vi "ParameterSubUI.vi"() -> ()   [LabVIEW 2016]
uses:
  Package ResourceControl/ViHandler/ViHandler.ViInfo.ctl
  Package Libraries/Message Queue/private/MessageQueue.MessageTypeDef.ctl
  Package ResourceControl/ViHandler/ViHandler.RunModes.ctl
  Package ErrorHandling/ErrorHandling.lvclass/ErrorHandling.ctl
  Package ErrorHandling/ErrorHandling.checkForErrorAndHandle.vi
  Package ErrorHandling/ErrorHandling.GetErrorHandler.vi
  <vilib>/Utility/error.llb/Clear Errors.vi
  Package Libraries/StringFunctions/StringFunctions_ReplaceAllBlindSigns.vi
  <vilib>/dlg_ctls.llb/Space Constant.vi
  Package Simulation/Modell/Umgebung/Umgebung.ParameterUI.vi
  Package Simulation/Modell/Hausmodell/Hausmodell.ParameterUI.vi
  <vilib>/Utility/error.llb/Error Cluster From Error Code.vi
  Package Libraries/TimingFunctions/TimingFunctions_getUtcTimestamp.vi
  <vilib>/Utility/error.llb/Trim Whitespace.vi
  <vilib>/Utility/error.llb/Search and Replace Pattern.vi
  Package ErrorHandling/ErrorHandling.addLastErrorToFile.vi
  <vilib>/ErrorRing/Error Ring.xnode
  Package ErrorHandling/ErrorHandling.lvclass
  Package ResourceControl/ViHandler/ViHandler.lvclass
  Package Simulation/Modell/Hausmodell/Hausmodell.lvclass
  Package Simulation/Modell/Sondenmodell/Sondenmodell.lvclass
  Package Simulation/Modell/Umgebung/Umgebung.lvclass
panel:
  in  "UmgebungBtn":bool
  in  "WPBtn":bool
  in  "SondenBtn":bool
  in  "HausBtn":bool
  out "EndOfBuffer[ms]":u32
  out "ViInfoTemp":T1
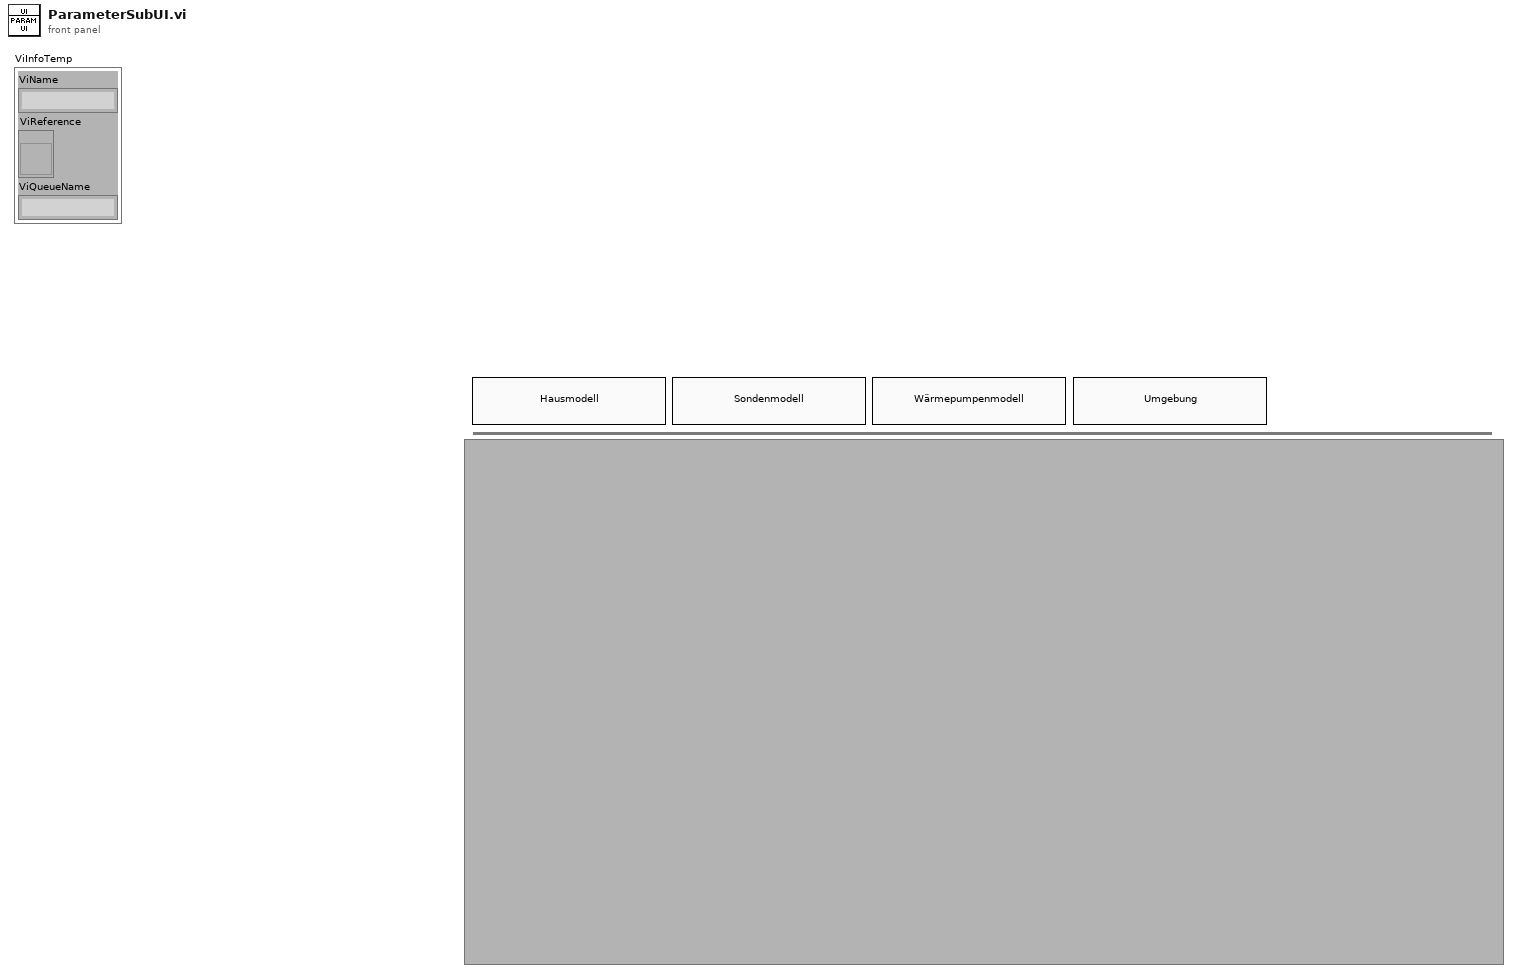
[diagram p1: front panel]
types:
  T1 = typedef "ViHandler.lvclass/ViHandler.ViInfo.ctl" = cluster{"ViName":string, "ViReference":refnum<vi>, "ViQueueName":string}
  T2 = typedef "MessageQueue.MessageTypeDef.ctl" = cluster{"Message":string, "Data":variant}
  T3 = typedef "ViHandler.lvclass/ViHandler.RunModes.ctl" = enum16{"FP Closed", "FP Open", "FP Open, Centered"}
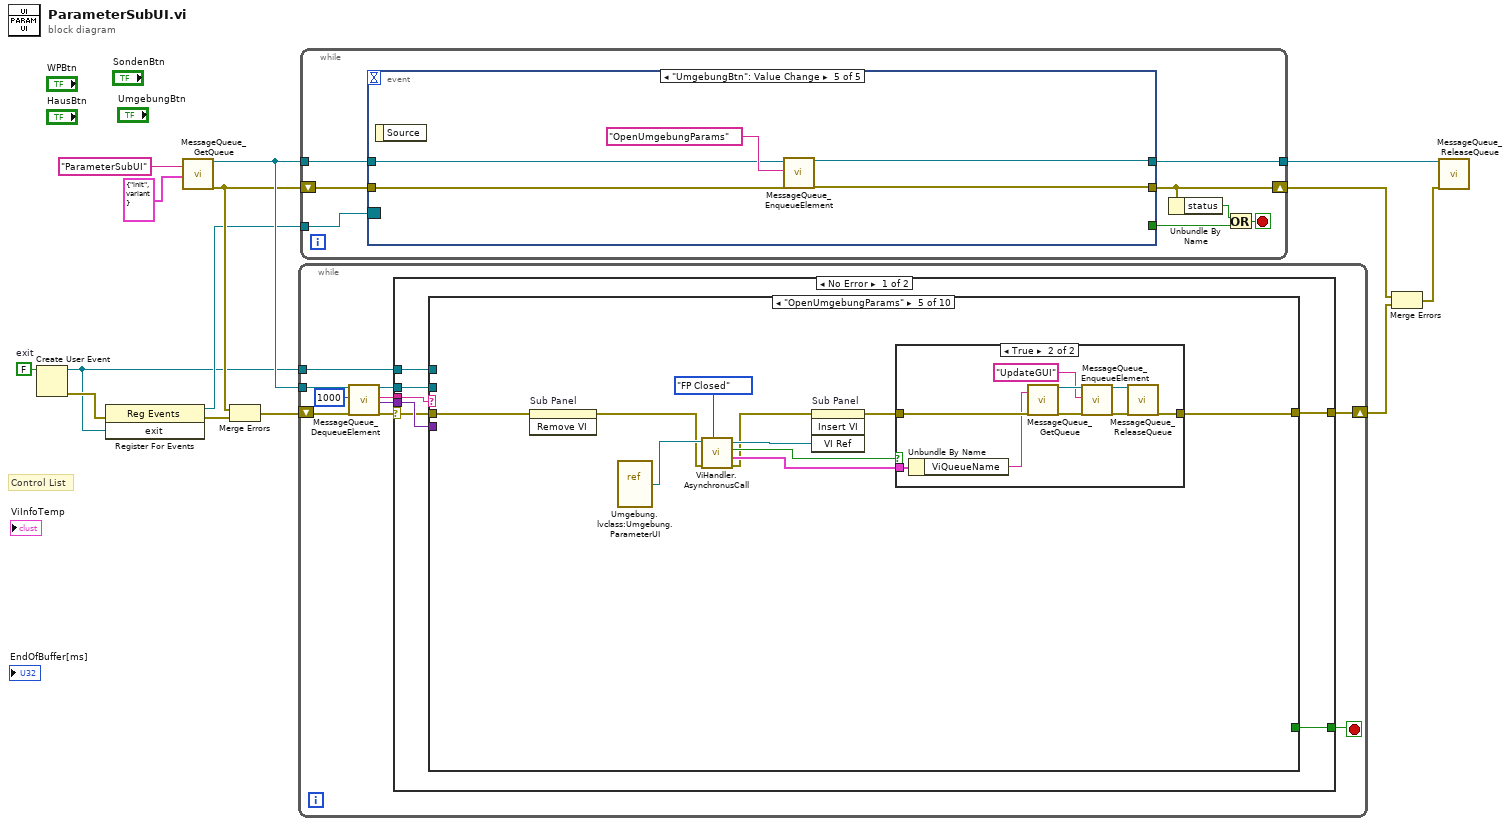
[diagram p0: block diagram]
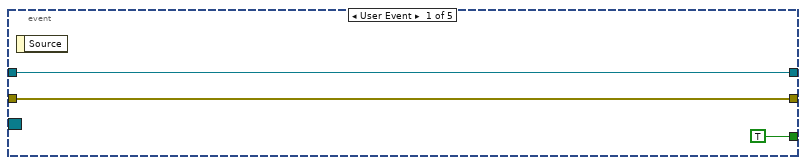
[diagram p2: hidden frame]
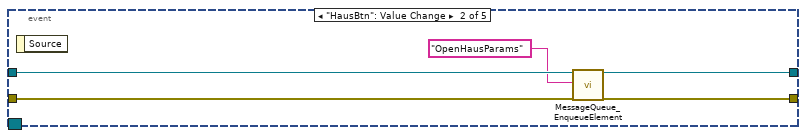
[diagram p3: hidden frame]
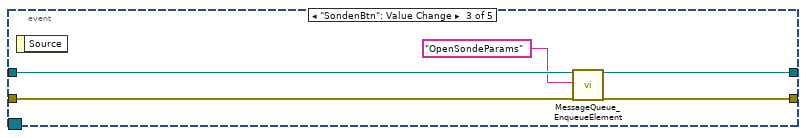
[diagram p4: hidden frame]
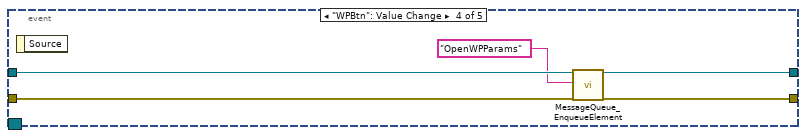
[diagram p5: hidden frame]
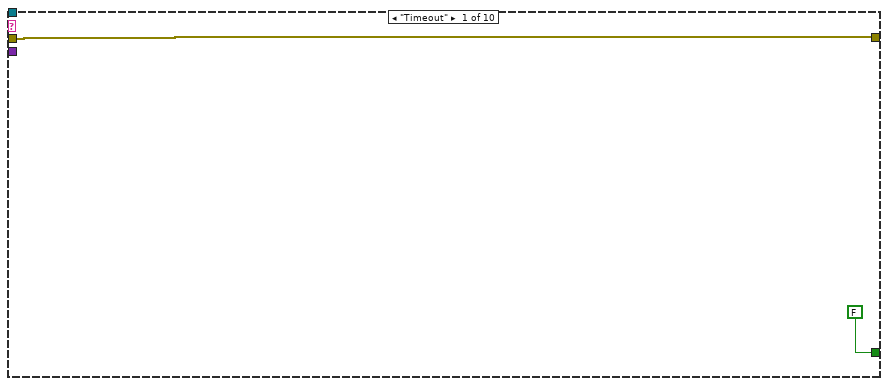
[diagram p6: hidden frame]
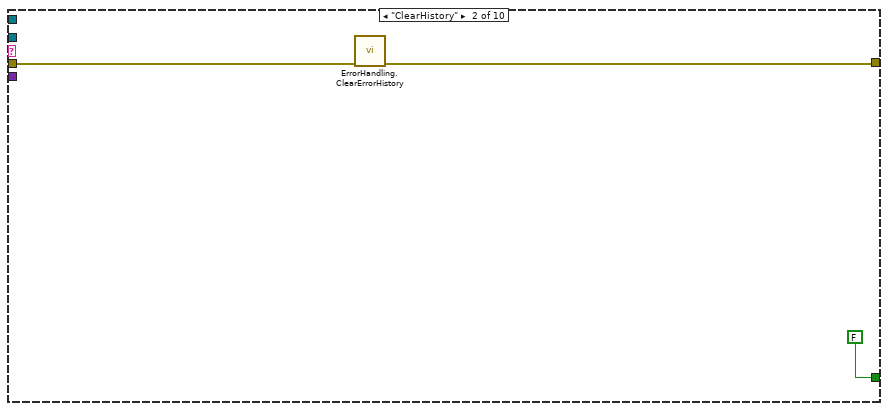
[diagram p7: hidden frame]
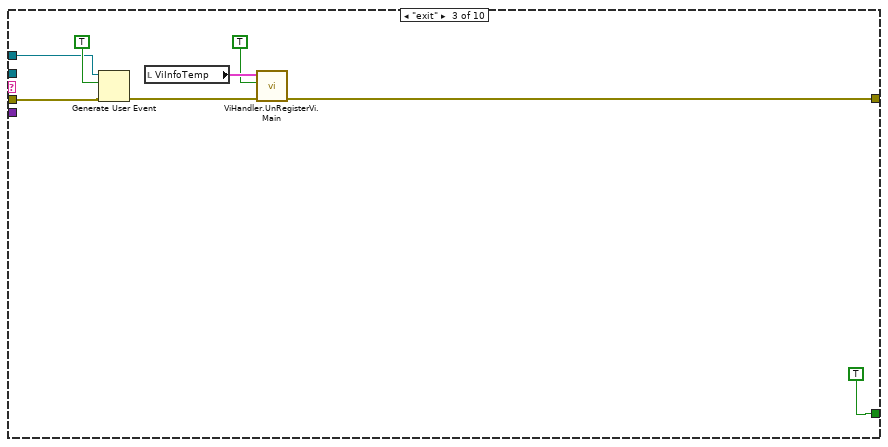
[diagram p8: hidden frame]
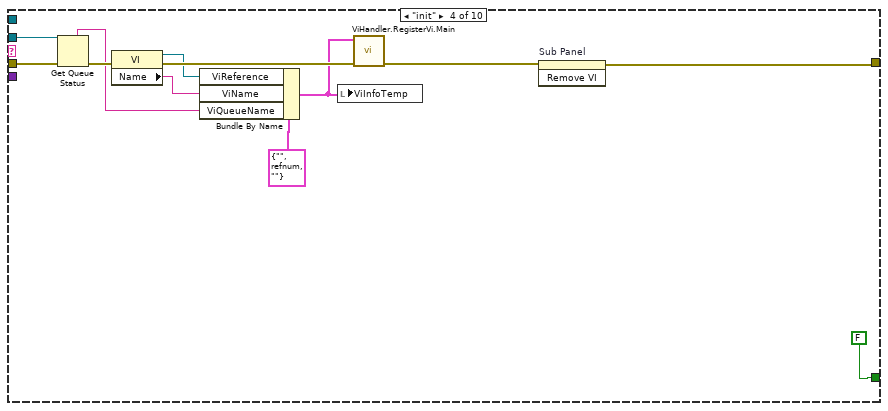
[diagram p9: hidden frame]
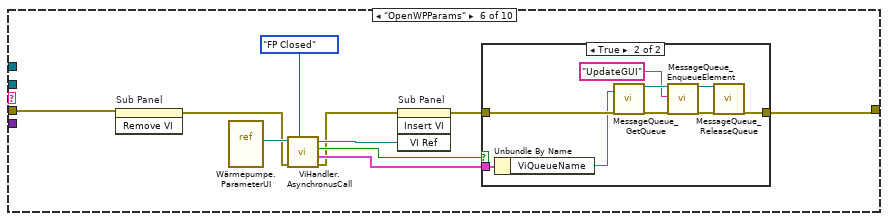
[diagram p11: hidden frame]
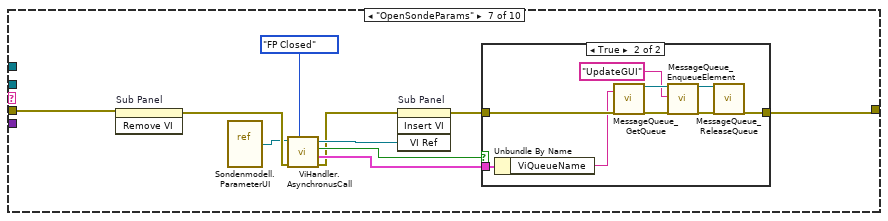
[diagram p13: hidden frame]
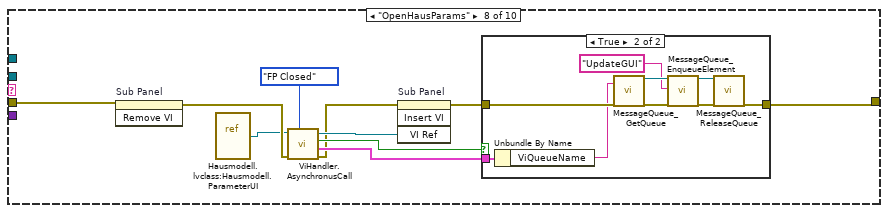
[diagram p15: hidden frame]
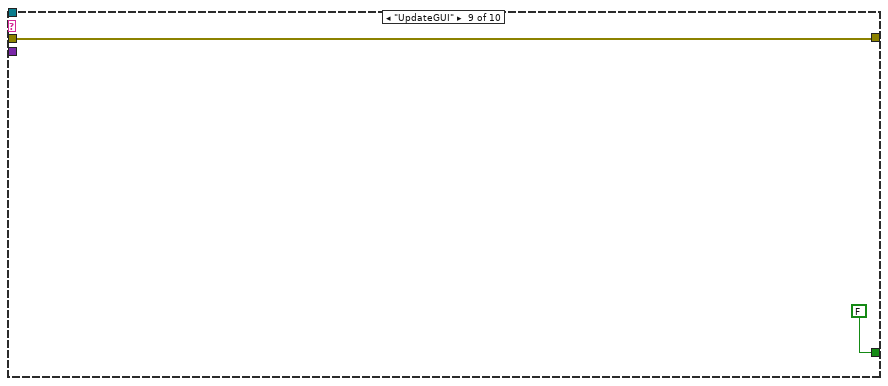
[diagram p17: hidden frame]
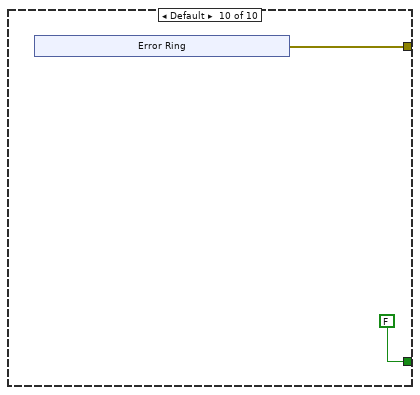
[diagram p18: hidden frame]
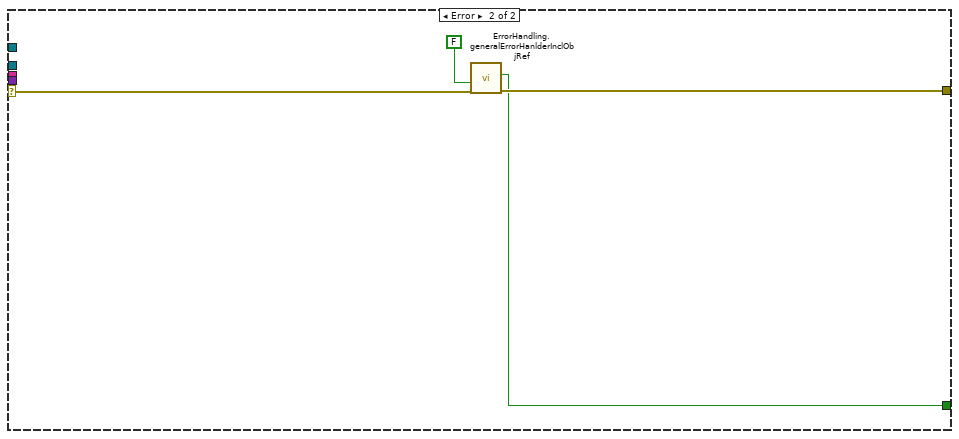
[diagram p19: hidden frame]
diagram:
  w7 = FALSE  # exit
  # "Control List"
  n1 = Create User Event(user event datatype=w7) -> (user event=w5:refnum<user-event>, error out=w6:errorcluster)  [unwired: 1 in]
  n2 = register-events(error in=w6, w5) -> (reference out=w9:refnum<event-registration>, error out=w11:errorcluster)  [unwired: 1 in]
  n3 = call "MessageQueue_GetQueue.vi"("Name"="ParameterSubUI", "OptionalInitValue"=T2 {"Message"="init", "Data"=variant}) -> ("QueueOut"=w13:refnum<queue>, "ErrorOut"=w10:errorcluster)  [unwired: 15 in, 1 out]
  n4 = Merge Errors(w10, w11) -> (w8:errorcluster)
  n5 = while {
    tunnel: w13 -> [w24]
    tunnel: w5 -> [w17]
    shift-right: [w16] -> w3
    shift-left: w8 -> [w18]
    stop <- w19 stop-if-true
    n6 = call "MessageQueue_DequeueElement.vi"("QueueIn"=w24, "Timeout"=1000, "ErrorIn"=w18) -> ("QueueOut"=w22:refnum<queue>, "Message"=w21:string, "Data"=w20:variant, "ErrorOut"=w23:errorcluster)  [unwired: 12 in, 1 out]
    n7 = case shown="No Error" w23 {
      selector: w23 -> [w27 w149]
      tunnel: w22 -> [w31 _]
      tunnel: w21 -> [w30 _]
      tunnel: w20 -> [w29 _]
      tunnel: [w28 w147] -> w19
      tunnel: w17 -> [w26 _]
      tunnel: [w25 w148] -> w16
      frame No Error {
        n8 = case shown="\"OpenUmgebungParams\"" w30 {
          tunnel: w31 -> [_ _ _ w50 _ _ _ _ _ _]
          tunnel: w29 -> [_ _ _ _ _ _ _ _ _ _]
          tunnel: [FALSE FALSE TRUE FALSE _ _ _ _ FALSE FALSE] -> w28
          tunnel: w27 -> [w32 w35 w42 w47 w58 w86 w106 w126 w137 _]
          tunnel: w26 -> [_ _ w41 _ _ _ _ _ _ _]
          tunnel: [w32 w34 w38 w45 w60 w79 w100 w120 w137 w140] -> w25
          frame "Timeout" {
          }
          frame "ClearHistory" {
            n9 = call "ErrorHandling.ClearErrorHistory.vi"("error IO"=w35) -> ("error IO"=w34:errorcluster)  [unwired: 10 in]
          }
          frame "exit" {
            n10 = Generate User Event(user event=w41, event data cluster=TRUE ("event data"), error in=w42) -> (error out=w39:errorcluster)  [unwired: 1 in, 1 out]
            n11 = local read "ViInfoTemp"() -> (w40:T1)
            n12 = call "ViHandler.UnRegisterVi.Main.vi"("ErrorIn"=w39, "FinalExit?"=TRUE, "ViInfo"=w40) -> ("ErrorOut"=w38:errorcluster)  [unwired: 7 in, 1 out]
          }
          frame "init" {
            n13 = Get Queue Status(queue=w50, error in (no error)=w47) -> (queue name=w48:string, error out=w54:errorcluster)  [unwired: 1 in, 6 out]
            n14 = property class="VI"(error in=w54) -> (reference out=w52:refnum<vi>, error out=w53:errorcluster, "Name"=w51:string)  [unwired: 1 in]
            n15 = Bundle By Name(cluster=T1 {"ViName"="", "ViReference"=refnum, "ViQueueName"=""} ("ViInfo"), "ViReference"=w52, "ViName"=w51, "ViQueueName"=w48) -> (w49:T1)
            n16 = local write "ViInfoTemp"(w49) -> ()
            n17 = call "ViHandler.RegisterVi.Main.vi"("ErrorIn"=w53, "ViInfo"=w49) -> ("ErrorOut"=w46:errorcluster)  [unwired: 9 in]
            n18 = invoke on="Sub Panel" class="SubPnl" method="Remove VI"(error in=w46) -> (error out=w45:errorcluster)  [unwired: 2 in, 2 out]
          }
          frame "OpenUmgebungParams" {
            n19 = invoke on="Sub Panel" class="SubPnl" method="Remove VI"(error in=w58) -> (error out=w57:errorcluster)  [unwired: 2 in, 2 out]
            n20 = vi-ref "Umgebung.lvclass:Umgebung.ParameterUI.vi"() -> (w59:refnum<vi>)
            n21 = call "ViHandler.AsynchronusCall.vi"("Modes"=ViHandler.RunModes."FP Closed", "Error In"=w57, "ViReference"=w59) -> ("error out"=w61:errorcluster, "ViInfo(OnlyIfFound=true)"=w62:T1, "ViFound?"=w63:bool, "ViReference"=w66:refnum<vi>)  [unwired: 5 in]
            n22 = invoke on="Sub Panel" class="SubPnl" method="Insert VI"(error in=w61, "VI Ref"=w66) -> (error out=w64:errorcluster)  [unwired: 2 in, 3 out]
            n23 = case shown="True" w63 {
              tunnel: w64 -> [w67 w76]
              tunnel: [w67 w73] -> w60
              tunnel: w62 -> [_ w72]
              frame False {
              }
              frame True {
                n24 = Unbundle By Name(w72) -> ("ViQueueName"=w69:string)
                n25 = call "MessageQueue_GetQueue.vi"("Name"=w69, "ErrorIn"=w76) -> ("QueueOut"=w71:refnum<queue>, "ErrorOut"=w75:errorcluster)  [unwired: 15 in, 1 out]
                n26 = call "MessageQueue_EnqueueElement.vi"("QueueIn"=w71, "Message"="UpdateGUI", "ErrorIn"=w75) -> ("QueueOut"=w70:refnum<queue>, "ErrorOut"=w74:errorcluster)  [unwired: 15 in]
                n27 = call "MessageQueue_ReleaseQueue.vi"("QueueIn"=w70, "ErrorIn"=w74) -> ("ErrorOut"=w73:errorcluster)  [unwired: 15 in, 2 out]
              }
            }
          }
          frame "OpenWPParams" {
            n28 = invoke on="Sub Panel" class="SubPnl" method="Remove VI"(error in=w86) -> (error out=w78:errorcluster)  [unwired: 2 in, 2 out]
            n29 = vi-ref "Wärmepumpe.ParameterUI.vi"() -> (w84:refnum<vi>)
            n30 = call "ViHandler.AsynchronusCall.vi"("Modes"=ViHandler.RunModes."FP Closed", "Error In"=w78, "ViReference"=w84) -> ("error out"=w77:errorcluster, "ViInfo(OnlyIfFound=true)"=w80:T1, "ViFound?"=w81:bool, "ViReference"=w85:refnum<vi>)  [unwired: 5 in]
            n31 = invoke on="Sub Panel" class="SubPnl" method="Insert VI"(error in=w77, "VI Ref"=w85) -> (error out=w82:errorcluster)  [unwired: 2 in, 3 out]
            n32 = case shown="True" w81 {
              tunnel: w82 -> [w87 w96]
              tunnel: [w87 w93] -> w79
              tunnel: w80 -> [_ w92]
              frame False {
              }
              frame True {
                n33 = Unbundle By Name(w92) -> ("ViQueueName"=w89:string)
                n34 = call "MessageQueue_GetQueue.vi"("Name"=w89, "ErrorIn"=w96) -> ("QueueOut"=w91:refnum<queue>, "ErrorOut"=w95:errorcluster)  [unwired: 15 in, 1 out]
                n35 = call "MessageQueue_EnqueueElement.vi"("QueueIn"=w91, "Message"="UpdateGUI", "ErrorIn"=w95) -> ("QueueOut"=w90:refnum<queue>, "ErrorOut"=w94:errorcluster)  [unwired: 15 in]
                n36 = call "MessageQueue_ReleaseQueue.vi"("QueueIn"=w90, "ErrorIn"=w94) -> ("ErrorOut"=w93:errorcluster)  [unwired: 15 in, 2 out]
              }
            }
          }
          frame "OpenSondeParams" {
            n37 = invoke on="Sub Panel" class="SubPnl" method="Remove VI"(error in=w106) -> (error out=w99:errorcluster)  [unwired: 2 in, 2 out]
            n38 = vi-ref "Sondenmodell.ParameterUI.vi"() -> (w97:refnum<vi>)
            n39 = call "ViHandler.AsynchronusCall.vi"("Modes"=ViHandler.RunModes."FP Closed", "Error In"=w99, "ViReference"=w97) -> ("error out"=w98:errorcluster, "ViInfo(OnlyIfFound=true)"=w101:T1, "ViFound?"=w102:bool, "ViReference"=w105:refnum<vi>)  [unwired: 5 in]
            n40 = invoke on="Sub Panel" class="SubPnl" method="Insert VI"(error in=w98, "VI Ref"=w105) -> (error out=w103:errorcluster)  [unwired: 2 in, 3 out]
            n41 = case shown="True" w102 {
              tunnel: w103 -> [w107 w116]
              tunnel: [w107 w113] -> w100
              tunnel: w101 -> [_ w112]
              frame False {
              }
              frame True {
                n42 = Unbundle By Name(w112) -> ("ViQueueName"=w109:string)
                n43 = call "MessageQueue_GetQueue.vi"("Name"=w109, "ErrorIn"=w116) -> ("QueueOut"=w111:refnum<queue>, "ErrorOut"=w115:errorcluster)  [unwired: 15 in, 1 out]
                n44 = call "MessageQueue_EnqueueElement.vi"("QueueIn"=w111, "Message"="UpdateGUI", "ErrorIn"=w115) -> ("QueueOut"=w110:refnum<queue>, "ErrorOut"=w114:errorcluster)  [unwired: 15 in]
                n45 = call "MessageQueue_ReleaseQueue.vi"("QueueIn"=w110, "ErrorIn"=w114) -> ("ErrorOut"=w113:errorcluster)  [unwired: 15 in, 2 out]
              }
            }
          }
          frame "OpenHausParams" {
            n46 = invoke on="Sub Panel" class="SubPnl" method="Remove VI"(error in=w126) -> (error out=w119:errorcluster)  [unwired: 2 in, 2 out]
            n47 = vi-ref "Hausmodell.lvclass:Hausmodell.ParameterUI.vi"() -> (w117:refnum<vi>)
            n48 = call "ViHandler.AsynchronusCall.vi"("Modes"=ViHandler.RunModes."FP Closed", "Error In"=w119, "ViReference"=w117) -> ("error out"=w118:errorcluster, "ViInfo(OnlyIfFound=true)"=w121:T1, "ViFound?"=w122:bool, "ViReference"=w125:refnum<vi>)  [unwired: 5 in]
            n49 = invoke on="Sub Panel" class="SubPnl" method="Insert VI"(error in=w118, "VI Ref"=w125) -> (error out=w123:errorcluster)  [unwired: 2 in, 3 out]
            n50 = case shown="True" w122 {
              tunnel: w123 -> [w127 w136]
              tunnel: [w127 w133] -> w120
              tunnel: w121 -> [_ w132]
              frame False {
              }
              frame True {
                n51 = Unbundle By Name(w132) -> ("ViQueueName"=w129:string)
                n52 = call "MessageQueue_GetQueue.vi"("Name"=w129, "ErrorIn"=w136) -> ("QueueOut"=w131:refnum<queue>, "ErrorOut"=w135:errorcluster)  [unwired: 15 in, 1 out]
                n53 = call "MessageQueue_EnqueueElement.vi"("QueueIn"=w131, "Message"="UpdateGUI", "ErrorIn"=w135) -> ("QueueOut"=w130:refnum<queue>, "ErrorOut"=w134:errorcluster)  [unwired: 15 in]
                n54 = call "MessageQueue_ReleaseQueue.vi"("QueueIn"=w130, "ErrorIn"=w134) -> ("ErrorOut"=w133:errorcluster)  [unwired: 15 in, 2 out]
              }
            }
          }
          frame "UpdateGUI" {
          }
          frame Default {
            n55 = xnode "Error Ring"() -> ("error out"=w140:errorcluster)
          }
        }
      }
      frame Error {
        n56 = call "ErrorHandling.generalErrorHanlderInclObjRef.vi"("error in"=w149, "StopOnError"=FALSE) -> ("error out"=w148:errorcluster, "Stop"=w147:bool)  [unwired: 7 in, 1 out]
      }
    }
  }
  n57 = while {
    tunnel: w13 -> [w157]
    tunnel: [w156] -> w14
    shift-right: [w153] -> w2
    shift-left: w10 -> [w155]
    tunnel: w9 -> [w150]
    stop <- w152 stop-if-true
    n58 = event shown="[4] \"UmgebungBtn\": Value Change" {
      selector: w150 -> [_ _ _ _ _]
      dyn-events: _ -> [_ _ _ _ _]
      timeout: _ -> [_ _ _ _ _]
      tunnel: w157 -> [w159 w165 w170 w175 w179]
      tunnel: [w159 w164 w169 w174 w178] -> w156
      tunnel: [w158 w162 w167 w172 w176] -> w153
      tunnel: w155 -> [w158 w163 w168 w173 w177]
      tunnel: [TRUE _ _ _ _] -> w154
      event User Event {
        n59 = event-data() -> ()  [unwired: 1 in, 1 out]
      }
      event "HausBtn": Value Change {
        n60 = event-data() -> ()  [unwired: 1 in, 1 out]
        n61 = call "MessageQueue_EnqueueElement.vi"("QueueIn"=w165, "Message"="OpenHausParams", "ErrorIn"=w163) -> ("QueueOut"=w164:refnum<queue>, "ErrorOut"=w162:errorcluster)  [unwired: 15 in]
      }
      event "SondenBtn": Value Change {
        n62 = event-data() -> ()  [unwired: 1 in, 1 out]
        n63 = call "MessageQueue_EnqueueElement.vi"("QueueIn"=w170, "Message"="OpenSondeParams", "ErrorIn"=w168) -> ("QueueOut"=w169:refnum<queue>, "ErrorOut"=w167:errorcluster)  [unwired: 15 in]
      }
      event "WPBtn": Value Change {
        n64 = event-data() -> ()  [unwired: 1 in, 1 out]
        n65 = call "MessageQueue_EnqueueElement.vi"("QueueIn"=w175, "Message"="OpenWPParams", "ErrorIn"=w173) -> ("QueueOut"=w174:refnum<queue>, "ErrorOut"=w172:errorcluster)  [unwired: 15 in]
      }
      event "UmgebungBtn": Value Change {
        n66 = event-data() -> ()  [unwired: 1 in, 1 out]
        n67 = call "MessageQueue_EnqueueElement.vi"("QueueIn"=w179, "Message"="OpenUmgebungParams", "ErrorIn"=w177) -> ("QueueOut"=w178:refnum<queue>, "ErrorOut"=w176:errorcluster)  [unwired: 15 in]
      }
    }
    n68 = Unbundle By Name(w153) -> ("status"=w151:bool)
    n69 = Or(x=w151, y=w154) -> (x .or. y?=w152:bool)
  }
  n70 = Merge Errors(w2, w3) -> (w1:errorcluster)
  n71 = call "MessageQueue_ReleaseQueue.vi"("QueueIn"=w14, "ErrorIn"=w1) -> ()  [unwired: 15 in, 3 out]
